vi "Configure Curve Header.vi"(0 "VISA resource name":refnum<visa-resource-name>, 1 "Curve Data Format (3: Ohms/K)":u16(ring)=3 items=["Ohms/K (Linear)"=3, "Log Ohms/K (Linear)"=4, "Ohms/K (Cubic Spline)"=7], 2 "Limit Value (0.000)":dbl min=0.0 max=1500.0 step=0.001 format="%.3f", 5 "Curve (21)":i32=21 min=21 max=59 step=1, 7 "Curve Name (\"\")":string, 9 "Curve Serial Number (\"\")":string, 11 "error in (no error)":errorcluster, 12 "Temp Coefficient (1: Negative)":u16(ring)=1 items=["Negative"=1, "Positive"=2]) -> (4 "VISA resource name out":refnum<visa-resource-name>, 15 "error out":errorcluster)   [LabVIEW 2015, in "Lake Shore 372.lvlib"]
doc: "Configures a user curve header.\n\nNote:\nThe coefficient parameter will be calculated automatically based on the first 2 curve datapoints."
uses:
  <instrlib>/Lake Shore 372/Lake Shore 372.lvlib
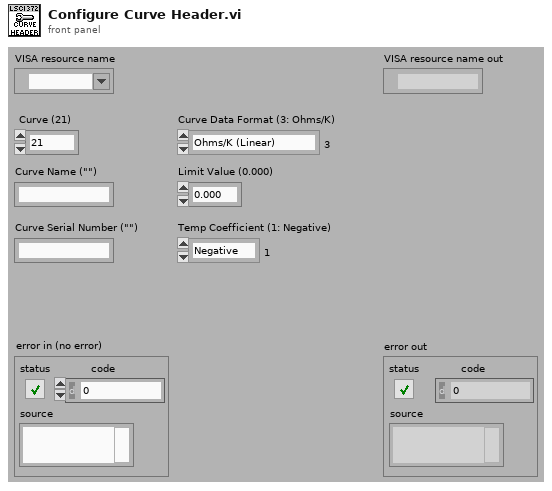
[diagram p1: front panel]
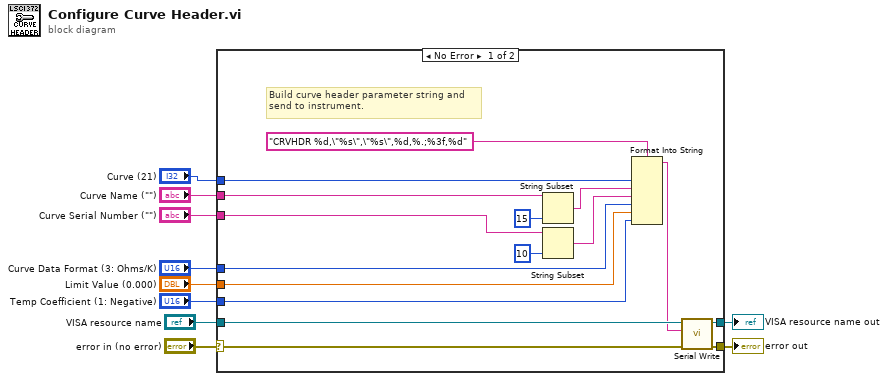
[diagram p0: block diagram]
diagram:
  n1 = case shown="No Error" "error in (no error)" {
    selector: "error in (no error)" -> [w17 w27]
    tunnel: "VISA resource name" -> [w24 w28]
    tunnel: [w23 w27] -> w9
    tunnel: [w22 w28] -> w8
    tunnel: "Curve (21)" -> [w16 _]
    tunnel: "Curve Name (\"\")" -> [w15 _]
    tunnel: "Curve Serial Number (\"\")" -> [w14 _]
    tunnel: "Curve Data Format (3: Ohms/K)" -> [w13 _]
    tunnel: "Limit Value (0.000)" -> [w12 _]
    tunnel: "Temp Coefficient (1: Negative)" -> [w11 _]
    frame No Error {
      # "Build curve header parameter string and\nsend to instrument."
      n2 = String Subset(string=w15, length (rest)=15) -> (substring=w20:string)  [unwired: 1 in]
      n3 = String Subset(string=w14, length (rest)=10) -> (substring=w19:string)  [unwired: 1 in]
      n4 = Format Into String(format string="CRVHDR %d,\"%s\",\"%s\",%d,%.;%3f,%d", w16, w20, w19, w13, w12, w11) -> (resulting string=w18:string)  [unwired: 2 in, 1 out]
      n5 = call <instrlib>:"Serial Write.vi"("error in (no error)"=w17, "Write Buffer (\"\")"=w18, "VISA resource name"=w24) -> ("error out"=w23:errorcluster, "VISA resource name out"=w22:refnum<visa-resource-name>)  [unwired: 6 in, 1 out]
    }
    frame Error {
    }
  }
  "error out" <- w9
  "VISA resource name out" <- w8
